vi "Build Preview for Rate.vi"(6 "Average During Loop ?":bool, 8 "error in (no error)":errorcluster, 9 "Loop ?":cluster{i32, i32}, 10 "Program":T1(array[cluster]), 11 "# Of Loops":u32) -> (0 "error out":errorcluster, 1 "Measure ? Out":bool[](array[boolean]), 2 "Y Values Out":dbl[](array[numeric]), 3 "Storage Locations Out":i32[](array[numeric]), 4 "Direction Out":bool[](array[boolean]), 5 "Plots Out":cluster{dbl[], dbl[]}[](array[cluster]), 7 "Stage Values":i32[](array[numeric]))   [LabVIEW 2018, in "Multi Segment Waveform.xctl"]
doc: "Builds a set of X-Y plots based on the current program and loop settings ."
uses:
  Multi Segment Waveform.xctl
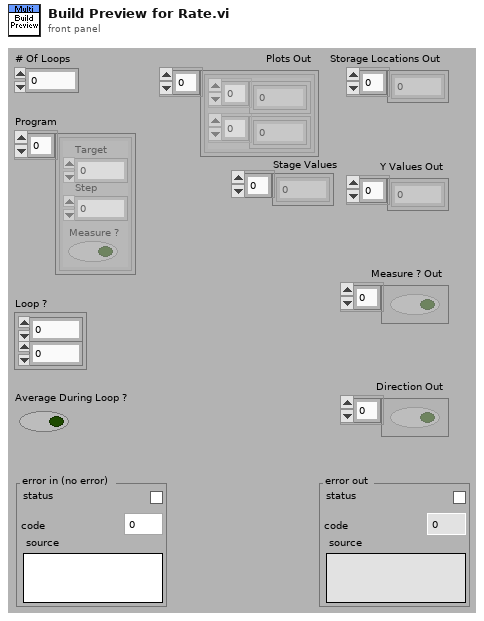
[diagram p1: front panel]
types:
  T1 = cluster{"Target":dbl, "Step":dbl, "Measure ?":bool}[]
  T2 = cluster{"Storage Locs":i32[], "Measure":bool[], "Field":dbl[], "Direction":bool[]}
  T3 = cluster{"Target":dbl, "Step":dbl, "Measure ?":bool}
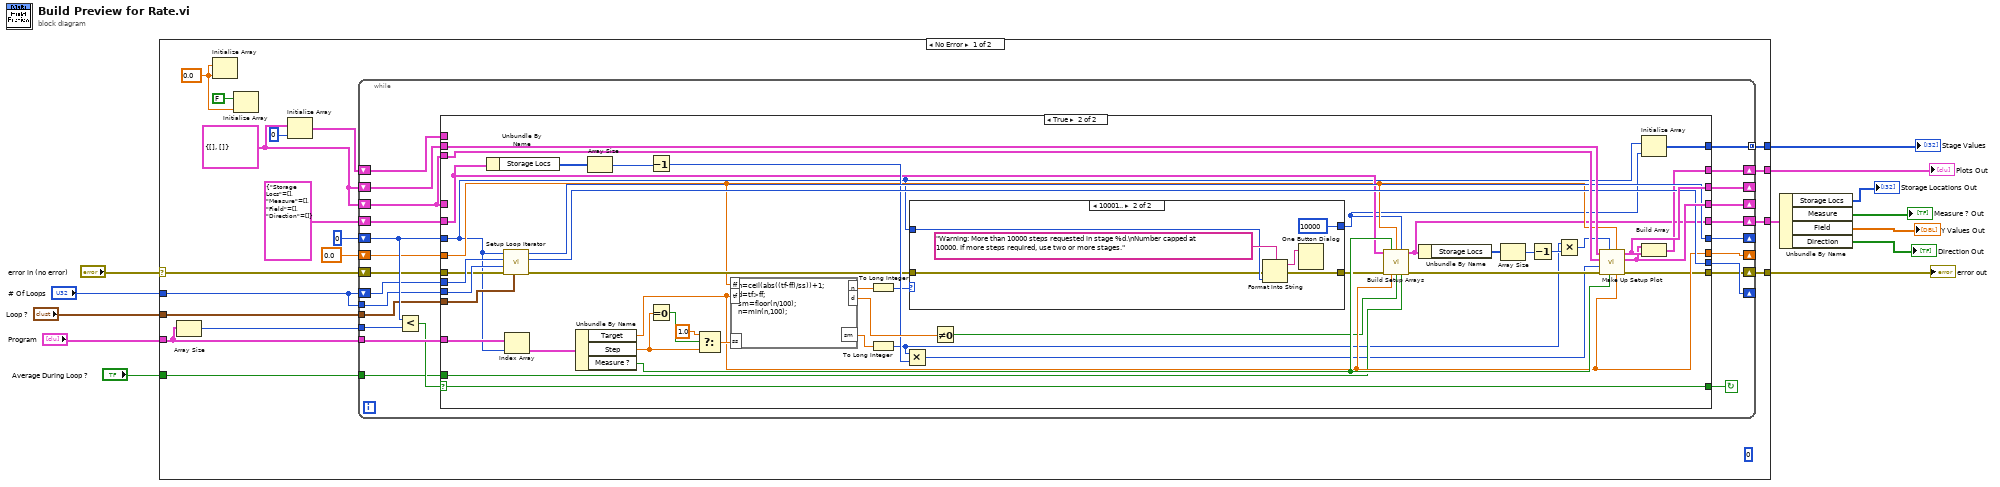
[diagram p0: block diagram]
diagram:
  n1 = case shown="No Error" "error in (no error)" {
    selector: "error in (no error)" -> [w17 w118]
    tunnel: [w28 _] -> w13
    tunnel: "Average During Loop ?" -> [w27 _]
    tunnel: "Loop ?" -> [w26 _]
    tunnel: "Program" -> [w25 _]
    tunnel: "# Of Loops" -> [w20 _]
    tunnel: [w18 _] -> w8
    tunnel: [w16 w118] -> w6
    tunnel: [w15 _] -> w5
    frame No Error {
      w29 = cluster{dbl[], dbl[]} {[], []}
      w19 = 0.0
      (unwired) 0
      n2 = Array Size(array=w25) -> (size(s)=w23:i32)
      n3 = Initialize Array(w19, w19) -> ()  [unwired: 1 out]
      n4 = Initialize Array(FALSE, w19) -> ()  [unwired: 1 out]
      n5 = Initialize Array(w29, 0 ("dimension size")) -> (w30:cluster{dbl[], dbl[]}[])
      n6 = while {
        shift-left: T2 {"Storage Locs"=[], "Measure"=[], "Field"=[], "Direction"=[]} ("Preview Out") -> [w40]
        shift-right: [w39] -> w18
        tunnel: w20 -> [w41]
        shift-left: w29 -> [w45]
        shift-right: [w44] -> _
        shift-left: w29 -> [w42]
        shift-right: [w43] -> _
        shift-left: w20 -> [w50]
        shift-right: [w49] -> _
        tunnel: w23 -> [w53]
        shift-left: 0 -> [w55]
        shift-right: [w48] -> _
        shift-left: 0.0 -> [w47]
        shift-right: [w46] -> _
        tunnel: w25 -> [w54]
        tunnel: w26 -> [w38]
        tunnel: w27 -> [w36]
        shift-right: [w37] -> w28
        shift-left: w30 -> [w35]
        shift-right: [w34] -> w16
        shift-left: w17 -> [w33]
        tunnel: [w32] -> w15 mode=concatenating
        stop <- w51 continue-if-true
        n7 = Less?(x=w55, y=w53) -> (x < y?=w52:bool)
        n8 = case shown="True" w52 {
          selector: w52 -> [w64 w99]
          tunnel: w55 -> [w62 w73]
          tunnel: w54 -> [_ w109]
          tunnel: [w64 w99] -> w51
          tunnel: w50 -> [w63 w102]
          tunnel: [w63 w101] -> w49
          tunnel: [w62 w100] -> w48
          tunnel: w47 -> [w61 w79]
          tunnel: [w61 w84] -> w46
          tunnel: w42 -> [_ w105]
          tunnel: w45 -> [w59 w104]
          tunnel: [w59 w107] -> w44
          tunnel: [w60 w106] -> w43
          tunnel: w42 -> [w60 _]
          tunnel: w41 -> [_ w103]
          tunnel: w40 -> [w58 w85]
          tunnel: [w58 w70] -> w39
          tunnel: w38 -> [_ w83]
          tunnel: [w57 w91] -> w37
          tunnel: w36 -> [_ w77]
          tunnel: w35 -> [w57 _]
          tunnel: [w56 w75] -> w34
          tunnel: w33 -> [w56 w82]
          tunnel: [_ w72] -> w32
          frame False {
          }
          frame True {
            n9 = Unbundle By Name(w85) -> ("Storage Locs"=w71:i32[])
            n10 = call "Setup Loop Iterator.vi"("Loop"=w83, "error in (no error)"=w82, "Total Loops"=w103, "Loop Iterator"=w102, "Previous Line"=w73) -> ("error out"=w81:errorcluster, "Loop Iterator Out"=w101:u32, "Line Iterator Out"=w100:i32)  [unwired: 4 out]
            n11 = Index Array(array=w109, index=w73) -> (element=w108:T3)
            n12 = Unbundle By Name(w108) -> ("Target"=w84:dbl, "Step"=w88:dbl, "Measure ?"=w92:bool)
            n13 = Array Size(array=w71) -> (size(s)=w94:i32)
            n14 = Decrement(x=w94) -> (x-1=w93:i32)
            n15 = Equal To 0?(x=w88) -> (x = 0?=w90:bool)
            n16 = Select(t=1.0, s=w90, f=w88) -> (s? t:f=w87:dbl)
            n17 = formula code="n=ceil(abs((tf-ff)/ss))+1;\nd=tf>ff;\nsm=floor(n/100);\nn=min(n,100);"("ff"=w79, "tf"=w84, "ss"=w87) -> ("n"=w97:dbl, "d"=w98:dbl, "sm"=w67:dbl)
            n18 = To Long Integer(number=w97) -> (32bit integer=w86:i32)
            n19 = To Long Integer(number=w67) -> (32bit integer=w65:i32)
            n20 = Multiply(x=w65, y=w93) -> (x*y=w68:i32)
            n21 = case shown="10001.." w86 {
              selector: w86 -> [w111 _]
              tunnel: [w111 10000] -> w74
              tunnel: w73 -> [_ w115]
              tunnel: w81 -> [w110 w113]
              tunnel: [w110 w112] -> w80
              frame ..10000 {
              }
              frame 10001.. {
                n22 = Format Into String(format string="Warning: More than 10000 steps requested in stage %d.\nNumber capped at 10000. If more steps required, use two or more stages.", error in=w113, w115) -> (resulting string=w114:string, error out=w112:errorcluster)  [unwired: 1 in]
                n23 = One Button Dialog(message=w114) -> ()  [unwired: 2 out]
              }
            }
            n24 = Not Equal To 0?(x=w98) -> (x != 0?=w78:bool)
            n25 = call "Build Setup Arrays.vi"("Preview In"=w85, "Measure ?"=w92, "First Field"=w79, "N Points"=w74, "error in (no error)"=w80, "Last Field"=w84, "Direction"=w78, "Average During Loop ?"=w77) -> ("Preview Out"=w70:T2, "error out"=w76:errorcluster)  [unwired: 3 in, 3 out]
            n26 = Unbundle By Name(w70) -> ("Storage Locs"=w69:i32[])
            n27 = Array Size(array=w69) -> (size(s)=w96:i32)
            n28 = Decrement(x=w96) -> (x-1=w95:i32)
            n29 = Multiply(x=w65, y=w95) -> (x*y=w66:i32)
            n30 = call "Make Up Setup Plot.vi"("End Field"=w84, "Start Field"=w79, "Put in plot 1"=w92, "End X"=w66, "error in (no error)"=w76, "Start X"=w68, "Plot 1 In"=w105, "Plot 2 In"=w104) -> ("error out"=w75:errorcluster, "Plot 1 Out"=w106:cluster{dbl[], dbl[]}, "Plot 2 Out"=w107:cluster{dbl[], dbl[]})  [unwired: 1 out]
            n31 = Initialize Array(w73, w74) -> (w72:i32[])
            n32 = Build Array(w106, w107) -> (w91:cluster{dbl[], dbl[]}[])
          }
        }
      }
    }
    frame Error {
    }
  }
  "Plots Out" <- w13
  "error out" <- w6
  "Stage Values" <- w5
  n33 = Unbundle By Name(w8) -> ("Storage Locs"=→"Storage Locations Out":i32[], "Measure"=→"Measure ? Out":bool[], "Field"=→"Y Values Out":dbl[], "Direction"=→"Direction Out":bool[])
